vi "8753ES_Save Data.vi"(2 "Step":string, 3 "Cap(pF)":dbl, 4 "Annotation Text Array":string[](array[string]), 5 "Cap Data File Path":path, 6 "Comment":string="K71382.8", 7 "C_min(pF)":dbl, 8 "error in":errorcluster, 9 "DeltaC Target(pF)":dbl, 10 "Wafer":string="W12", 11 "Lot":string="K71382.8") -> (0 "error out":errorcluster, 1 "% Delta C":dbl)   [LabVIEW 2009]
panel:
  in  "Cap Data -Header":string[][](table)
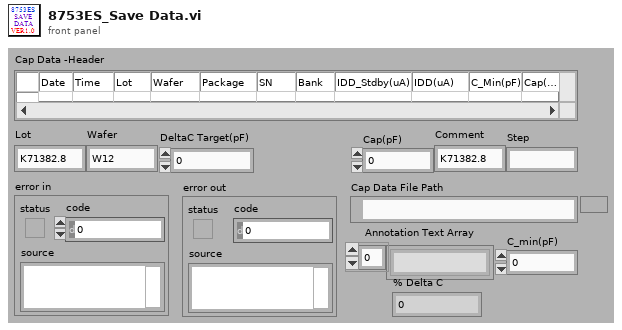
[diagram p1: front panel]
types:
  T1 = enum16{"open", "replace", "create", "open or create", "replace or create", "replace or create with confirmation"}
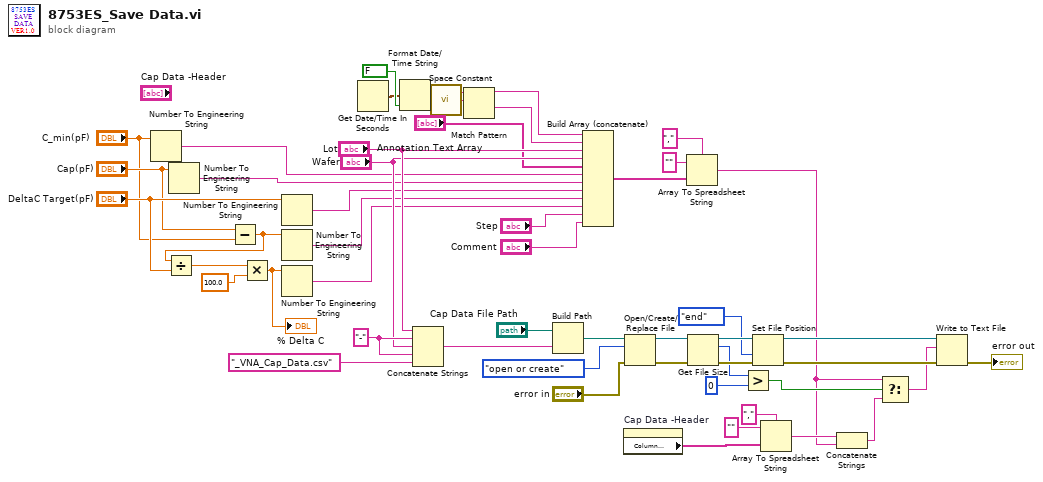
[diagram p0: block diagram]
diagram:
  w19 = "-"
  n1 = Number To Engineering String(4:"C_min(pF)") -> (0:w4:string)  [unwired: 1 in, 2 out]
  n2 = Number To Engineering String(4:"Cap(pF)") -> (0:w5:string)  [unwired: 1 in, 2 out]
  n3 = Subtract(x="Cap(pF)", y="C_min(pF)") -> (x-y=w1:dbl)
  n4 = Divide(x=w1, y="DeltaC Target(pF)") -> (x/y=w14:dbl)
  n5 = Multiply(x=w14, y=100.0) -> (x*y=w12:dbl)
  "% Delta C" <- w12
  n6 = Number To Engineering String(4:"DeltaC Target(pF)") -> (0:w6:string)  [unwired: 1 in, 2 out]
  n7 = Number To Engineering String(4:w1) -> (0:w7:string)  [unwired: 1 in, 2 out]
  n8 = Number To Engineering String(4:w12) -> (0:w8:string)  [unwired: 1 in, 2 out]
  n9 = Get Date/Time In Seconds() -> (seconds since 1Jan1904=w31:timestamp)
  n10 = Format Date/Time String(seconds (now)=w31, UTC format=FALSE) -> (date/time string=w33:string)  [unwired: 1 out]
  n11 = Concatenate Strings("Lot", w19, "Wafer", w19, "_VNA_Cap_Data.csv" ("string")) -> (w25:string)
  n12 = call <vilib>:"Space Constant.vi"() -> ("String"=w36:string)
  n13 = Match Pattern(string=w33, regular expression=w36) -> (before substring=w34:string, after substring=w35:string)  [unwired: 3 out]
  n14 = Build Path(base path="Cap Data File Path", name or relative path=w25) -> (appended path=w23:path)
  n15 = Build Array (concatenate)(w34, w35, "Lot", "Wafer", "Annotation Text Array", w4, w5, w6, w7, w8, "Step", "Comment") -> (w22:string[])
  n16 = property on="Cap Data -Header" class="Tbl (strict)"() -> ("Column Headers[]"=w37:string[])  [unwired: 2 in, 2 out]
  n17 = Open/Create/Replace File(file path (use dialog)=w23, error in="error in", operation (0:open)=T1."open or create") -> (refnum out=w51:refnum<file>, error out=w46:errorcluster)  [unwired: 4 out]
  n18 = Array To Spreadsheet String(delimiter (Tab)=",", array=w22, 3:"" ("format string")) -> (spreadsheet string=w29:string)
  n19 = Get File Size(file=w51, error in=w46) -> (refnum out=w50:refnum<file>, size (in bytes)=w45:i64, 0:w48:errorcluster)
  n20 = Greater?(x=w45, y=i64 0) -> (0:w42:bool)
  n21 = Set File Position(refnum=w50, from (0:start)=enum16{"start", "end", "current"}."end", error in=w48) -> (refnum out=w49:refnum<file>, error out=w47:errorcluster)  [unwired: 1 out]
  n22 = Array To Spreadsheet String(delimiter (Tab)=",", array=w37, 3:"" ("format string")) -> (spreadsheet string=w41:string)
  n23 = Concatenate Strings(w41, w29) -> (w27:string)
  n24 = Select(t=w29, s=w42, f=w27) -> (s? t:f=w39:string)
  n25 = Write to Text File(file (use dialog)=w49, text=w39, error in=w47) -> (error out=→"error out":errorcluster)  [unwired: 3 out]
